vi "Compute Decay & Time Gates.vi"(6 "Version":enum32{"Version 1", "Version 2"}(radio), 8 "Error In":errorcluster, 9 "Decay & Gates Options":T3, 10 "Gates Definitions":T6={"First Gate: t1"=0.0, "Gate Width: W"=4.0, "Gate Step: d"=0.3, "# Gates: G"=50.0, "Use Gate Center"=FALSE, "Frames/Image: F"=50, "Gates/Frame: L"=0, "Bits/Frame: q"=0, "Multiplicity: p"=0, "Gate Type"=enum."Square", "Gate Edge s"=4.0, "Gate Top Slope"=4.0, "Reversed Sawtooth?"=FALSE, "Computation"=FALSE, "User-defined Gate"={"X Array"=[], "Y Array"=[]}, "Tolerance"=50.0, "Integration"=enum."Item 0", "# Steps"=50.0, "Type of User-defined Function"=enum."Gate"}, 11 "Decay Definition":T4={"offset: t0"=2.0, "period: T"=15.0, "lifetime: tau"=0.5, "Incident Signal: I"=0.5, "Normalized Decays"=FALSE, "IRF Model"=enum."Dirac", "IRF Parameter 1"=0.0, "Poisson Signal"=FALSE}) -> (0 "Error Out":errorcluster, 1 "Gate Sum":dbl, 2 "Plot Names":string[](array[string]), 3 "Plots":cluster{"t Array":dbl[], "Gate Array":dbl[]}[](array[cluster]), 4 "Decay Analysis Results":T1 {"A" format="%#_5g"; "tau" format="%#_5g"; "Bkgd" format="%#_5g"; "Min" format="%#_5g"; "Max" format="%#_5g"}, 5 "Scales":cluster{"X Scale":u32, "Y Scale":u32}[](array[cluster]), 7 "Plots Interpolation (Previous Plot's Style)":T2[](array[typedef]) items=["Point (.)", "Stepwise Right (--.)", "Line + Point (\\. /)", "Stepwise Left (.--)", "Stepwise Centered (-.-)", "Stepwise Vertical (|.|)", "Line (-)", "Use Previous Plot's Style"])   [LabVIEW 2019]
uses:
  Gate Definitions.ctl
  Gate Type.ctl
  Graphs/XY Graph/XY Plot Data.ctl
  Decay Definiton.ctl
  IRF Model.ctl
  Decay & Gates Options.ctl
  Graphs/LabVIEW Plot Interpolation.ctl
  Gate Analysis Results.ctl
  Arrays/Linear Ramp End Options.ctl
  8f995b8f-6563-4a36-b24f-17447402644a.vi/69b89faf-335b-4e54-b1eb-c494efef2307.vi
  Square Gated 1-Exp Parameters.ctl
  <vilib>/gmath/NI_Gmath.lvlib
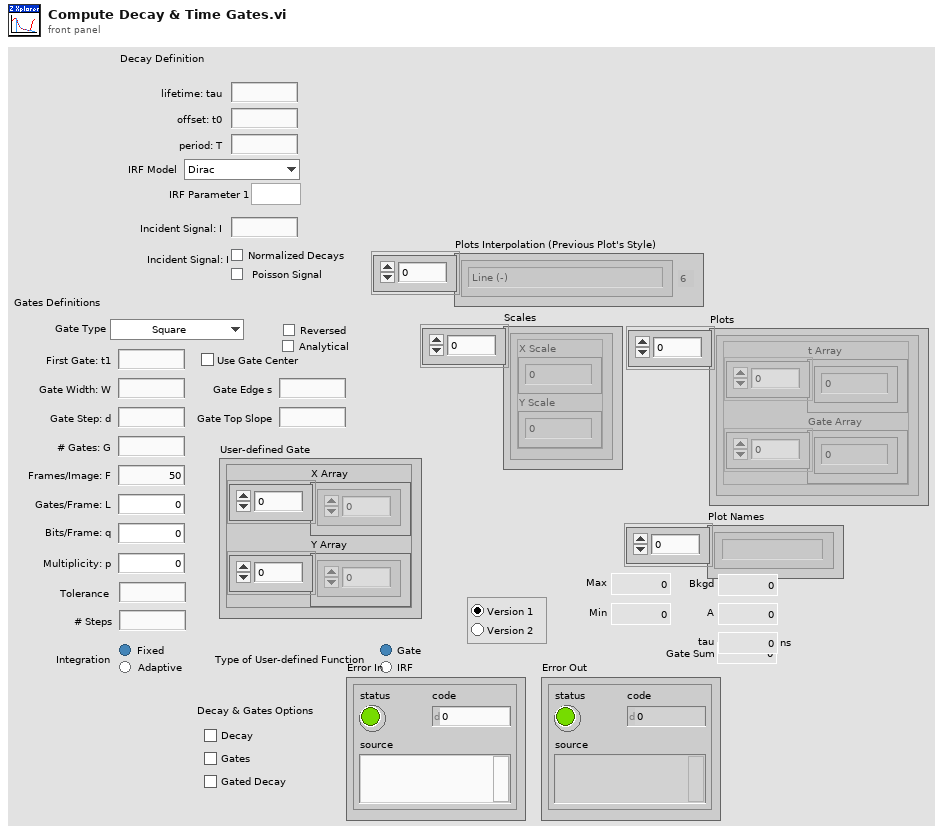
[diagram p1: front panel]
types:
  T1 = typedef "Gate Analysis Results.ctl" = cluster{"Max":dbl, "Min":dbl, "Bkgd":dbl, "tau ":dbl[unit], "A":dbl}
  T2 = typedef "LabVIEW Plot Interpolation.ctl" = u8
  T3 = typedef "Decay & Gates Options.ctl" = cluster{"Decay":bool, "Gate":bool, "Gated Decay":bool}
  T4 = typedef "Decay Definiton.ctl" = cluster{"offset: t0":ext, "period: T":ext, "lifetime: tau":ext, "Incident Signal: I":ext, "Normalized Decays":bool, "IRF Model":T5, "IRF Parameter 1":ext, "Poisson Signal":bool}
  T5 = typedef "IRF Model.ctl" = enum16{"Dirac", "Exponential"}
  T6 = typedef "Gate Definitions.ctl" = cluster{"First Gate: t1":ext, "Gate Width: W":ext, "Gate Step: d":ext, "# Gates: G":ext, "Use Gate Center":bool, "Frames/Image: F":i32, "Gates/Frame: L":i32, "Bits/Frame: q":i32, "Multiplicity: p":i32, "Gate Type":T7, "Gate Edge s":ext, "Gate Top Slope":ext, "Reversed Sawtooth?":bool, "Computation":bool, "User-defined Gate":T8, "Tolerance":ext, "Integration":enum32{"Item 0", "Item 1"}, "# Steps":ext, "Type of User-defined Function":enum32{"Gate", "IRF"}}
  T7 = typedef "Gate Type.ctl" = enum16{"Square", "Finite Edge Square", "Finite Edge, Tilted Top Square", "Triangle", "Sawtooth", "User-defined"}
  T8 = typedef "XY Plot Data.ctl" = cluster{"X Array":dbl[], "Y Array":dbl[]}
  T9 = typedef "Linear Ramp End Options.ctl" = enum16{"Include Min/Exclude Max", "Exclude Min/Include Max", "Include Both Ends", "Exclude Both Ends"}
  T10 = cluster{"Ramp":ext[], "Poisson Randomized Array":ext[]}
  T11 = typedef "Square Gated 1-Exp Parameters.ctl" = cluster{"P-R":dbl, "W":dbl, "T":dbl}
  T12 = cluster{"t Array":ext[], "Gate Image Array":ext[]}
  T13 = cluster{"t Array":ext[], "Gate Image Array":ext[]}[]
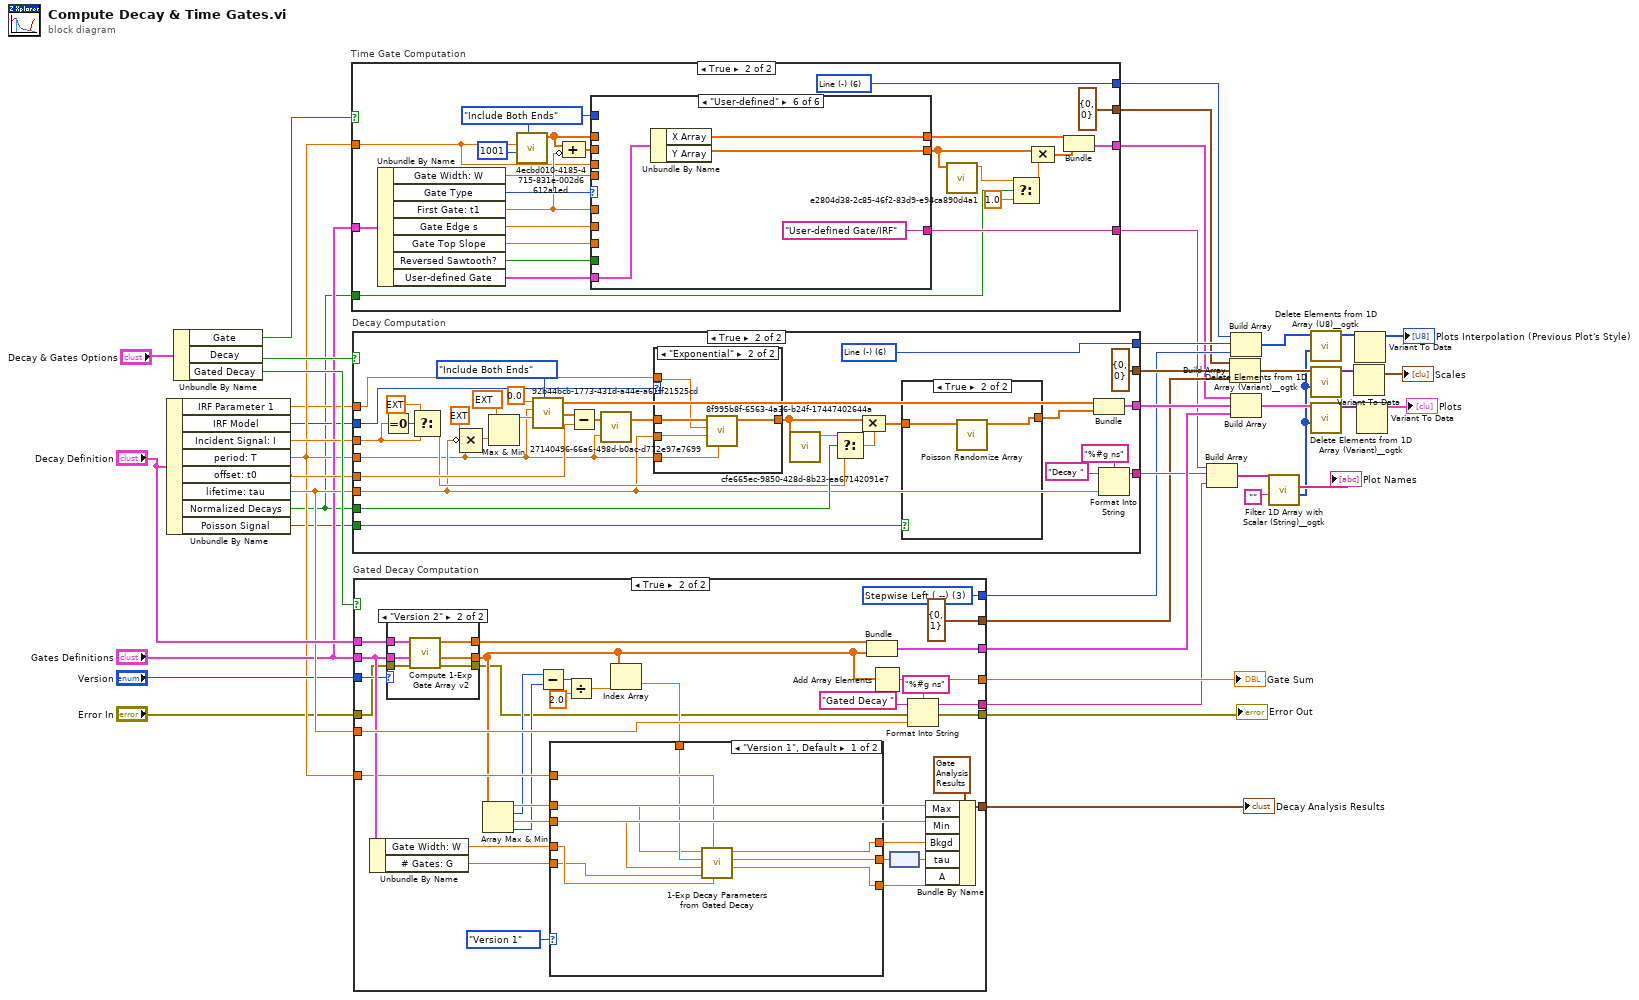
[diagram p0: block diagram]
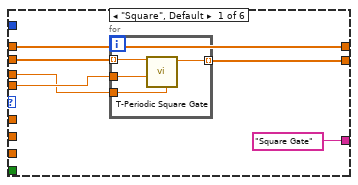
[diagram p3: hidden frame]
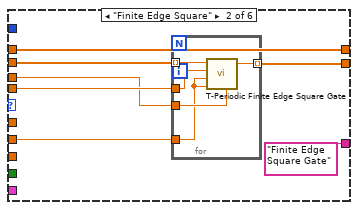
[diagram p4: hidden frame]
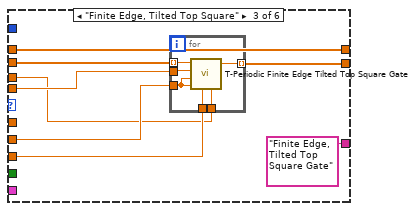
[diagram p5: hidden frame]
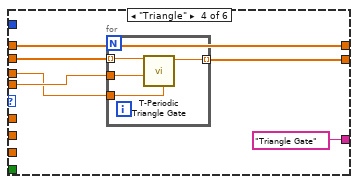
[diagram p6: hidden frame]
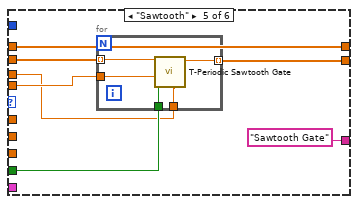
[diagram p7: hidden frame]
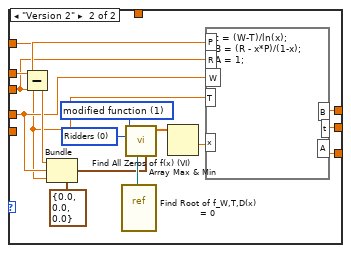
[diagram p9: hidden frame]
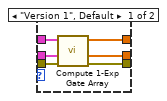
[diagram p10: hidden frame]
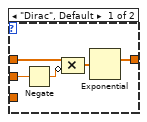
[diagram p13: hidden frame]
diagram:
  n1 = Unbundle By Name("Decay Definition") -> ("IRF Parameter 1"=w5:ext, "IRF Model"=w6:T5, "Incident Signal: I"=w14:ext, "period: T"=w7:ext, "offset: t0"=w17:ext, "lifetime: tau"=w36:ext, "Normalized Decays"=w1:bool, "Poisson Signal"=w2:bool)
  n2 = Unbundle By Name("Decay & Gates Options") -> ("Gate"=w13:bool, "Decay"=w40:bool, "Gated Decay"=w39:bool)
  n3 = case "Time Gate Computation" shown="True" w13 {
    tunnel: [_ w68] -> w9
    tunnel: [_ cluster{"X Scale":u32, "Y Scale":u32} {"X Scale"=0, "Y Scale"=0} ("Cluster")] -> w10
    tunnel: [_ w66] -> w11
    tunnel: "Gates Definitions" -> [_ w65]
    tunnel: [_ w63] -> w8
    tunnel: w7 -> [_ w51]
    tunnel: w1 -> [_ w49]
    frame False {
    }
    frame True {
      w66 = T2 6 items=["Point (.)", "Stepwise Right (--.)", "Line + Point (\\. /)", "Stepwise Left (.--)", "Stepwise Centered (-.-)", "Stepwise Vertical (|.|)", "Line (-)", "Use Previous Plot's Style"] ("Plots Interpolation (Previous Plot's Style)")
      w58 = Linear_Ramp_End_Options."Include Both Ends" ("Options")
      n4 = Unbundle By Name(w65) -> ("Gate Width: W"=w57:ext, "Gate Type"=w64:T7, "First Gate: t1"=w62:ext, "Gate Edge s"=w61:ext, "Gate Top Slope"=w60:ext, "Reversed Sawtooth?"=w53:bool, "User-defined Gate"=w52:T8)
      n5 = call "4ecbd010-4185-4715-831e-002d6612a1ed.vi"("Options"=w58, "# Steps (1)"=1001 ("# Steps"), "End (1)"=w51) -> ("Ramp"=w55:ext[])  [unwired: 6 in, 2 out]
      n6 = Compound Arithmetic op=ADD(w55, invert w62) -> (w56:ext[])
      n7 = case shown="\"User-defined\"" w64 {
        tunnel: w56 -> [w73 w81 w93 w109 w120 _]
        tunnel: w62 -> [_ _ _ _ _ _]
        tunnel: [w71 w84 w97 w107 w118 w127] -> w50
        tunnel: ["Square Gate" "Finite Edge Square Gate" "Finite Edge, Tilted Top Square Gate" "Triangle Gate" "Sawtooth Gate" "User-defined Gate/IRF"] -> w63
        tunnel: w57 -> [w72 w82 w95 w108 w119 _]
        tunnel: w61 -> [_ w83 w94 _ _ _]
        tunnel: w60 -> [_ _ w96 _ _ _]
        tunnel: w58 -> [_ _ _ _ _ _]
        tunnel: w55 -> [w70 w80 w92 w106 w117 _]
        tunnel: [w70 w80 w92 w106 w117 w129] -> w54
        tunnel: w53 -> [_ _ _ _ w116 _]
        tunnel: w52 -> [_ _ _ _ _ w128]
        tunnel: w51 -> [w69 w79 w91 w105 w115 _]
        frame "Square", Default {
          n8 = for {
            tunnel: w73 -> [w78] mode=indexing
            tunnel: w72 -> [w77]
            tunnel: [w76] -> w71 mode=indexing
            tunnel: w69 -> [w75]
            n9 = call "T-Periodic Square Gate.vi"("Period T"=w75, "W"=w77, "t"=w78) -> ("Square(t)"=w76:dbl)  [unwired: 8 in]
          }
        }
        frame "Finite Edge Square" {
          n10 = for {
            tunnel: [w90] -> w84 mode=indexing
            tunnel: w82 -> [w89]
            tunnel: w83 -> [w86]
            tunnel: w81 -> [w88] mode=indexing
            tunnel: w79 -> [w87]
            n11 = call "T-Periodic Finite Edge Square Gate.vi"("Period T"=w87, "s_F"=w86, "s_R"=w86, "W"=w89, "t"=w88) -> ("Finite Edge Square(t)"=w90:dbl)  [unwired: 6 in]
          }
        }
        frame "Finite Edge, Tilted Top Square" {
          n12 = for {
            tunnel: [w104] -> w97 mode=indexing
            tunnel: w95 -> [w103]
            tunnel: w94 -> [w101]
            tunnel: w96 -> [w100]
            tunnel: w93 -> [w102] mode=indexing
            tunnel: w91 -> [w99]
            n13 = call "T-Periodic Finite Edge Tilted Top Square Gate.vi"("Period T"=w99, "slope"=w100, "s_F"=w101, "s_R"=w101, "W"=w103, "t"=w102) -> ("Finite Edge Square(t)"=w104:dbl)  [unwired: 5 in]
          }
        }
        frame "Triangle" {
          n14 = for {
            tunnel: w109 -> [w114] mode=indexing
            tunnel: w108 -> [w113]
            tunnel: [w112] -> w107 mode=indexing
            tunnel: w105 -> [w111]
            n15 = call "T-Periodic Triangle Gate.vi"("Period T"=w111, "W"=w113, "t"=w114) -> ("Triangle(t)"=w112:dbl)  [unwired: 8 in]
          }
        }
        frame "Sawtooth" {
          n16 = for {
            tunnel: w120 -> [w126] mode=indexing
            tunnel: w119 -> [w125]
            tunnel: [w124] -> w118 mode=indexing
            tunnel: w116 -> [w123]
            tunnel: w115 -> [w122]
            n17 = call "T-Periodic Sawtooth Gate.vi"("Period T"=w122, "Reversed?"=w123, "W"=w125, "t"=w126) -> ("Sawtooth(t)"=w124:dbl)  [unwired: 7 in]
          }
        }
        frame "User-defined" {
          n18 = Unbundle By Name(w128) -> ("X Array"=w129:dbl[], "Y Array"=w127:dbl[])
        }
      }
      n19 = call "e2804d38-2c85-46f2-83d9-e94ca890d4a1.vi"("y(t)"=w50) -> ("Peak Normalization Factor"=w48:dbl)  [unwired: 10 in]
      n20 = Select(t=w48, s=w49, f=1.0) -> (s? t:f=w45:dbl)
      n21 = Compound Arithmetic op=MULTIPLY(w50, w45) -> (w46:dbl[])
      n22 = Bundle("Ramp"=w54, w46) -> (w68:cluster{"Ramp":ext[], dbl[]})  [unwired: 1 in]
    }
  }
  n23 = case "Decay Computation" shown="True" w40 {
    tunnel: [_ w159] -> w44
    tunnel: [_ w153] -> w38
    tunnel: w36 -> [_ w142]
    tunnel: [_ cluster{"X Scale":u32, "Y Scale":u32} {"X Scale"=0, "Y Scale"=0} ("Cluster")] -> w28
    tunnel: [_ w151] -> w23
    tunnel: w7 -> [_ w135]
    tunnel: w17 -> [_ w150]
    tunnel: w14 -> [_ w147]
    tunnel: w1 -> [_ w146]
    tunnel: w6 -> [_ w137]
    tunnel: w5 -> [_ w136]
    tunnel: w2 -> [_ w133]
    frame False {
    }
    frame True {
      w151 = T2 6 items=["Point (.)", "Stepwise Right (--.)", "Line + Point (\\. /)", "Stepwise Left (.--)", "Stepwise Centered (-.-)", "Stepwise Vertical (|.|)", "Line (-)", "Use Previous Plot's Style"] ("Plots Interpolation (Previous Plot's Style)")
      n24 = Equal To 0?(x=w147) -> (x = 0?=w149:bool)
      n25 = Select(t=ext 1.0, s=w149, f=w147) -> (s? t:f=w145:ext)
      n26 = Compound Arithmetic op=MULTIPLY(ext 10.0 ("value"), invert w142, w135) -> (w140:ext)
      n27 = Max & Min(x=ext 1001.0, y=w140) -> (max(x,y)=w138:ext)  [unwired: 1 out]
      n28 = call "92b44bcb-1773-431d-a44e-a61ff21525cd.vi"("Options"=Linear_Ramp_End_Options."Include Both Ends", "# Steps (1)"=w138, "End (1)"=w135, "Start (0)"=0.0 ("Min")) -> ("Ramp"=w160:ext[])  [unwired: 5 in, 2 out]
      n29 = Subtract(x=w160, y=w150) -> (x-y=w157:ext[])
      n30 = call "27140496-66a6-498d-b0ac-d772e97e7699.vi"("y"=w135, "x"=w157) -> ("x - E(x/y)y"=w156:ext[])  [unwired: 1 out]
      n31 = case shown="\"Exponential\"" w137 {
        tunnel: w156 -> [w169 w174]
        tunnel: [w166 w170] -> w134
        tunnel: w142 -> [w165 w172]
        tunnel: w136 -> [_ w173]
        tunnel: w135 -> [_ w171]
        frame "Dirac", Default {
          n32 = Negate(x=w165) -> (-x=w168:ext)
          n33 = Compound Arithmetic op=MULTIPLY(w169, invert w168) -> (w167:ext[])
          n34 = Exponential(1:w167) -> (0:w166:ext[])
        }
        frame "Exponential" {
          n35 = call "8f995b8f-6563-4a36-b24f-17447402644a.vi"("Period: T"=w171, "lifetime: tau"=w172, "IRF time constant"=w173, "t"=w174) -> ("y(t)"=w170:ext[])  [unwired: 6 in, 1 out]
        }
      }
      n36 = call "cfe665ec-9850-428d-8b23-ea67142091e7.vi"("y(t)"=w134) -> ("Peak Normalization Factor"=w143:ext)  [unwired: 10 in]
      n37 = Select(t=w143, s=w146, f=w145) -> (s? t:f=w144:ext)
      n38 = Compound Arithmetic op=MULTIPLY(w134, w144) -> (w132:ext[])
      n39 = case shown="True" w133 {
        tunnel: w132 -> [w162 w164]
        tunnel: [w162 w163] -> w131
        frame False {
        }
        frame True {
          n40 = call "Poisson Randomize Array.vi"("Array"=w164) -> ("Poisson Randomized Array"=w163:dbl[])  [unwired: 10 in]
        }
      }
      n41 = Bundle("Ramp"=w160, "Poisson Randomized Array"=w131) -> (w159:T10)  [unwired: 1 in]
      n42 = Format Into String(format string="%#g ns", initial string="Decay ", w142) -> (resulting string=w153:string)  [unwired: 1 in, 1 out]
    }
  }
  n43 = case "Gated Decay Computation" shown="True" w39 {
    tunnel: [_ w209] -> w43
    tunnel: "Decay Definition" -> [_ w208]
    tunnel: "Gates Definitions" -> [_ w201]
    tunnel: [_ w207] -> w42
    tunnel: w36 -> [_ w205]
    tunnel: [_ w204] -> w35
    tunnel: [_ cluster{"X Scale":u32, "Y Scale":i32} {"X Scale"=0, "Y Scale"=1} ("Cluster")] -> w27
    tunnel: [_ w202] -> w22
    tunnel: w7 -> [_ w192]
    tunnel: [_ w199] -> w16
    tunnel: "Version" -> [_ w183]
    tunnel: "Error In" -> [w175 w178]
    tunnel: [w175 w176] -> w3
    frame False {
    }
    frame True {
      w202 = T2 3 items=["Point (.)", "Stepwise Right (--.)", "Line + Point (\\. /)", "Stepwise Left (.--)", "Stepwise Centered (-.-)", "Stepwise Vertical (|.|)", "Line (-)", "Use Previous Plot's Style"] ("Plots Interpolation (Previous Plot's Style)")
      n44 = Unbundle By Name(w201) -> ("Gate Width: W"=w193:ext, "# Gates: G"=w179:ext)
      n45 = case shown="\"Version 2\"" w183 {
        tunnel: w208 -> [w239 w245]
        tunnel: w201 -> [w238 w244]
        tunnel: [w237 w243] -> w190
        tunnel: [w236 w242] -> w185
        tunnel: [w234 w241] -> w177
        tunnel: w178 -> [w235 w240]
        frame "Version 1", Default {
          n46 = call "Compute 1-Exp Gate Array.vi"("Error In"=w235, "Gates Definitions"=w238, "Decay Definition"=w239) -> ("Error Out"=w234:errorcluster, "Gate Array"=w236:dbl[], "t Array"=w237:dbl[])  [unwired: 6 in]
        }
        frame "Version 2" {
          n47 = call "Compute 1-Exp Gate Array v2.vi"("Error In"=w240, "Gates Definitions"=w244, "Decay Definition"=w245) -> ("Error Out"=w241:errorcluster, "Gate Image Array"=w242:ext[], "t Array"=w243:ext[])  [unwired: 4 in, 2 out]
        }
      }
      n48 = Array Max & Min(array=w185) -> (max value=w198:ext, max index (indices)=w189:i32, min value=w197:ext, min index (indices)=w188:i32)
      n49 = Subtract(x=w189, y=w188) -> (x-y=w187:i32)
      n50 = Divide(x=w187, y=2.0) -> (x/y=w186:dbl)
      n51 = Index Array(array=w185, index=w186) -> (element=w184:ext)
      n52 = case shown="\"Version 1\", Default" enum32{"Version 1", "Version 2"}."Version 1" ("Version") {
        tunnel: w198 -> [w211 w226]
        tunnel: w197 -> [w213 w225]
        tunnel: [w218 w227] -> w196
        tunnel: [w217 w224] -> w195
        tunnel: w193 -> [w216 w223]
        tunnel: w192 -> [w215 w222]
        tunnel: w184 -> [w212 _]
        tunnel: [w214 w219] -> w180
        tunnel: w179 -> [w210 _]
        frame "Version 1", Default {
          n53 = call "1-Exp Decay Parameters from Gated Decay.vi"("Gate Width: W"=w216, "period: T"=w215, "# Gates"=w210, "Min Decay"=w213, "Mid Decay"=w212, "Max Decay"=w211) -> ("x"=w214:dbl, "tau"=w217:dbl, "B"=w218:dbl)  [unwired: 2 in, 1 out]
        }
        frame "Version 2" {
          w232 = u16 0 items=["Ridders", "Newton Raphson"] ("algorithm")
          w233 = u16 1 items=["fixed function", "modified function"] ("step type")
          n54 = Subtract(x=w226, y=w225) -> (x-y=w231:ext)
          n55 = Bundle(cluster=T11 {"P-R"=0.0, "W"=0.0, "T"=0.0} ("Square Gated Single Exponential Parameters"), "P-R"=w231, "W"=w223, "T"=w222) -> (w229:T11)
          n56 = vi-ref "Find Root of f_W,T,D(x) = 0.vi"() -> (w230:refnum<vi>)
          n57 = call <vilib>:"Find All Zeros of f(x) (VI).vi"("data"=w229, "f(x)"=w230, "algorithm"=w232, "step type"=w233) -> ("Zeros"=w228:dbl[])  [unwired: 4 in, 3 out]
          n58 = Array Max & Min(array=w228) -> (min value=w221:dbl)  [unwired: 3 out]
          n59 = formula code="t = (W-T)/ln(x);\nB = (R - x*P)/(1-x);\nA = 1;"("P"=w226, "R"=w225, "x"=w221, "W"=w223, "T"=w222) -> ("B"=w227:dbl, "t"=w224:dbl, "A"=w219:dbl)
        }
      }
      n60 = Bundle("t Array"=w190, "Gate Image Array"=w185) -> (w209:T12)  [unwired: 1 in]
      n61 = Add Array Elements(numeric array=w185) -> (sum=w207:ext)
      n62 = node(w195) -> (w194:dbl[unit])
      n63 = Format Into String(format string="%#g ns", initial string="Gated Decay ", error in=w177, w205) -> (resulting string=w204:string, error out=w176:errorcluster)
      n64 = Bundle By Name(cluster=T1 {"Max"=19.0, "Min"=19.0, "Bkgd"=19.0, "tau "=1.9e-08, "A"=0.0} ("Decay Analysis Results"), "Max"=w198, "Min"=w197, "Bkgd"=w196, "tau"=w194, "A"=w180) -> (w199:T1)
    }
  }
  "Gate Sum" <- w42
  "Error Out" <- w3
  "Decay Analysis Results" <- w16
  n65 = Build Array(w8, w38, w35) -> (w34:string[])
  n66 = Build Array(w10, w28, w27) -> (w26:cluster{"X Scale":u32, "Y Scale":u32}[])
  n67 = Build Array(w11, w23, w22) -> (w21:T2[])
  n68 = Build Array(w9, w44, w43) -> (w31:T13)
  n69 = call <userlib>:"Filter 1D Array with Scalar (String)__ogtk.vi"("items to filter"="", "array"=w34) -> ("filtered item indices"=w20:i32[], "filtered array"=→"Plot Names":string[])  [unwired: 4 in]
  n70 = call <userlib>:"Delete Elements from 1D Array (U8)__ogtk.vi"("indices"=w20, "array"=w21) -> ("array w/ subset deleted"=w19:u8[])  [unwired: 8 in, 1 out]
  n71 = call <userlib>:"Delete Elements from 1D Array (Variant)__ogtk.vi"("indices"=w20, "array"=w26) -> ("array w/ subset deleted"=w25:variant[])  [unwired: 8 in, 1 out]
  n72 = call <userlib>:"Delete Elements from 1D Array (Variant)__ogtk.vi"("indices"=w20, "array"=w31) -> ("array w/ subset deleted"=w30:variant[])  [unwired: 8 in, 1 out]
  n73 = Variant To Data(Variant=w25) -> (data=→"Scales":cluster{"X Scale":u32, "Y Scale":u32}[])  [unwired: 2 in, 1 out]
  n74 = Variant To Data(Variant=w19) -> (data=→"Plots Interpolation (Previous Plot's Style)":T2[])  [unwired: 2 in, 1 out]
  n75 = Variant To Data(Variant=w30) -> (data=→"Plots":cluster{"t Array":dbl[], "Gate Array":dbl[]}[])  [unwired: 2 in, 1 out]
